vi "Apply Highpass Filter.vi"(6 "Initial Filter State":dbl[](array[numeric]) format="%.2f", 8 "error in (no error)":errorcluster, 9 "init/cont (init:F)":bool, 10 "filter coefficients":T1 {"Forward Coefficients" format="%.4f"; "Reverse Coefficients" format="%.4f"}, 11 "signal [V]":waveform(sgl)={"t0"=timestamp(0 s since 1904-01-01), "dt"=0.0, "Y"=[]}) -> (0 "error out":errorcluster, 3 "filtered signal [EU]":waveform(sgl), 4 "Final Filter State":dbl[](array[numeric]) format="%.2f")   [LabVIEW 2017, in "VibrationAnalysisFunctions.lvlib"]
uses:
  <vilib>/addons/InsightCM/Utilities/Analysis/Vibration/VibrationAnalysisFunctions.lvlib
  <resource>/lvanlys.dll
  <vilib>/Analysis/NI_AALBase.lvlib
  <vilib>/Analysis/3filter.llb/IIR Cascade Filter with I.C. (DBL).vi
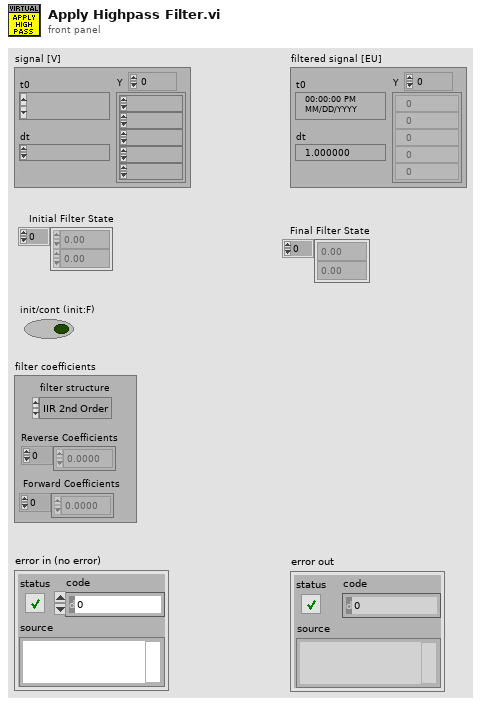
[diagram p1: front panel]
types:
  T1 = cluster{"filter structure":enum32{"IIR 2nd Order", "IIR 4th Order"}, "Reverse Coefficients":dbl[], "Forward Coefficients":dbl[]}
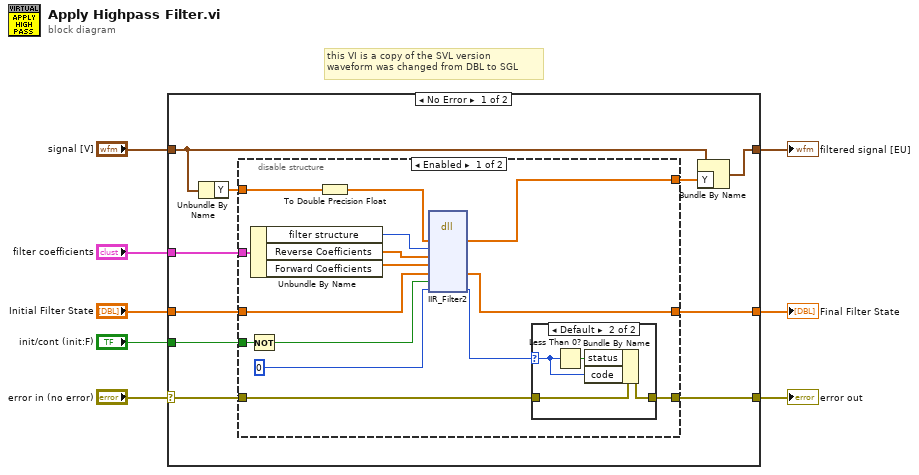
[diagram p0: block diagram]
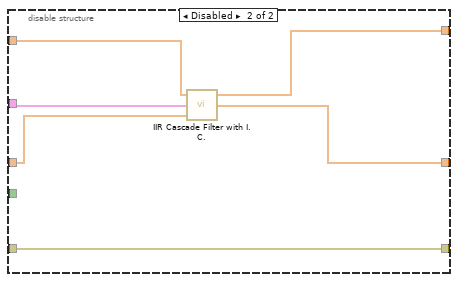
[diagram p3: hidden frame]
diagram:
  # "this VI is a copy of the SVL version\nwaveform was changed from DBL to SGL"
  n1 = case shown="No Error" "error in (no error)" {
    selector: "error in (no error)" -> [w13 w47]
    tunnel: "filter coefficients" -> [w15 _]
    tunnel: "signal [V]" -> [w18 w46]
    tunnel: [w17 w46] -> w6
    tunnel: [w12 w47] -> w1
    tunnel: "init/cont (init:F)" -> [w9 _]
    tunnel: "Initial Filter State" -> [w11 w45]
    tunnel: [w10 w45] -> w3
    frame No Error {
      n2 = Unbundle By Name(w18) -> ("Y"=w16:sgl[])
      n3 = disable-structure shown="Enabled" {
        disable-tunnel: w16 -> [w20 w44]
        disable-tunnel: w15 -> [w29 w42]
        disable-tunnel: [w28 w43] -> w14
        disable-tunnel: w9 -> [w26 _]
        disable-tunnel: w13 -> [w24 w39]
        disable-tunnel: [w23 w39] -> w12
        disable-tunnel: w11 -> [w22 w41]
        disable-tunnel: [w21 w40] -> w10
        frame Enabled {
          n4 = Not(x=w26) -> (.not. x?=w27:bool)
          n5 = Unbundle By Name(w29) -> ("filter structure"=w32:enum32{"IIR 2nd Order", "IIR 4th Order"}, "Reverse Coefficients"=w31:dbl[], "Forward Coefficients"=w30:dbl[])
          n6 = To Double Precision Float(number=w20) -> (double precision float=w19:dbl[])
          n7 = dll-call lib="C:/Program Files (x86)/National Instruments/LabVIEW 2017/resource/lvanlys.*" fn="IIR_Filter2"("Y"=w19, "filter structure"=w32, "Reverse Coefficients"=w31, "Forward Coefficients"=w30, "Initial Filter State"=w22, "output param"=w27, "output param"=0) -> ("Y"=w28:dbl[], "Initial Filter State"=w21:dbl[], "output param"=w25:i32)  [unwired: 8 in, 2 out]
          n8 = case shown="Default" w25 {
            selector: w25 -> [_ w35]
            tunnel: w24 -> [w34 w38]
            tunnel: [w34 w37] -> w23
            frame 0 {
            }
            frame Default {
              n9 = Less Than 0?(x=w35) -> (x < 0?=w36:bool)
              n10 = Bundle By Name(cluster=w38, "status"=w36, "code"=w35) -> (w37:errorcluster)
            }
          }
        }
        frame Disabled {
          n11 = call-poly <vilib>:"IIR Cascade Filter with I.C..vi"("Initial Filter State"=w41, "IIR Filter Cluster"=w42, "X"=w44) -> ("Final Filter State"=w40:dbl[], "Filtered X"=w43:dbl[])  [unwired: 1 out]
        }
      }
      n12 = Bundle By Name(cluster=w18, "Y"=w14) -> (w17:waveform(sgl))
    }
    frame Error {
    }
  }
  "filtered signal [EU]" <- w6
  "Final Filter State" <- w3
  "error out" <- w1
